vi "test Disconnect All.vi"(8 "error in (no error)":errorcluster, 11 "TestCase in":refnum<class "Switch Consumer Test Case.lvclass">) -> (0 "error out":errorcluster, 3 "TestCase out":refnum<class "Switch Consumer Test Case.lvclass">)   [LabVIEW 2017, in "Switch Consumer Test Case.lvclass"]
uses:
  Switch Consumer Test Case.lvclass
  Switch/Switch Disconnect All Message/Switch Disconnect All Message.lvclass
  C:/github/niveristand-custom-device-message-library/Source/Message/Abstract Message/Abstract Message.lvclass
  Support/Message String Action.ctl
  Switch Consumer Test Case.lvclass/Switch Consumer Test Case.ctl
  Producer/Abstract Producer/Abstract Producer.lvclass
  <vilib>/addons/_JKI Toolkits/VI Tester/TestCase.llb/TestCase.lvclass
  Consumer/Abstract Consumer/Abstract Consumer.lvclass
  C:/Program Files (x86)/National Instruments/LabVIEW 2017/vi.lib/addons/_JKI Toolkits/VI Tester/TestCase.llb/TestCase.lvclass
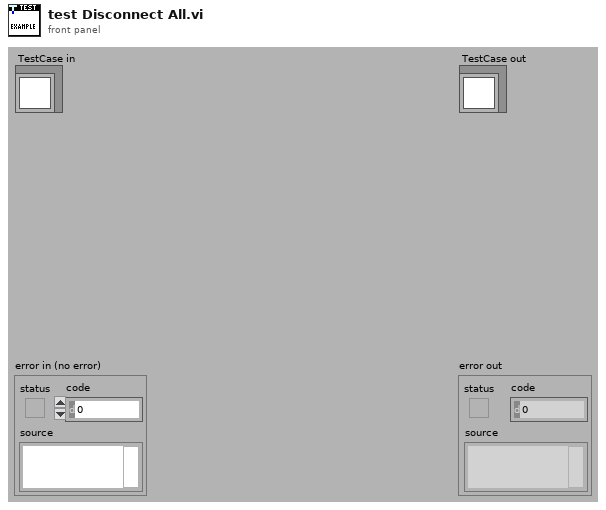
[diagram p1: front panel]
types:
  T1 = typedef "Message String Action.ctl" = enum16{"Get String", "Set String", "Reset"}
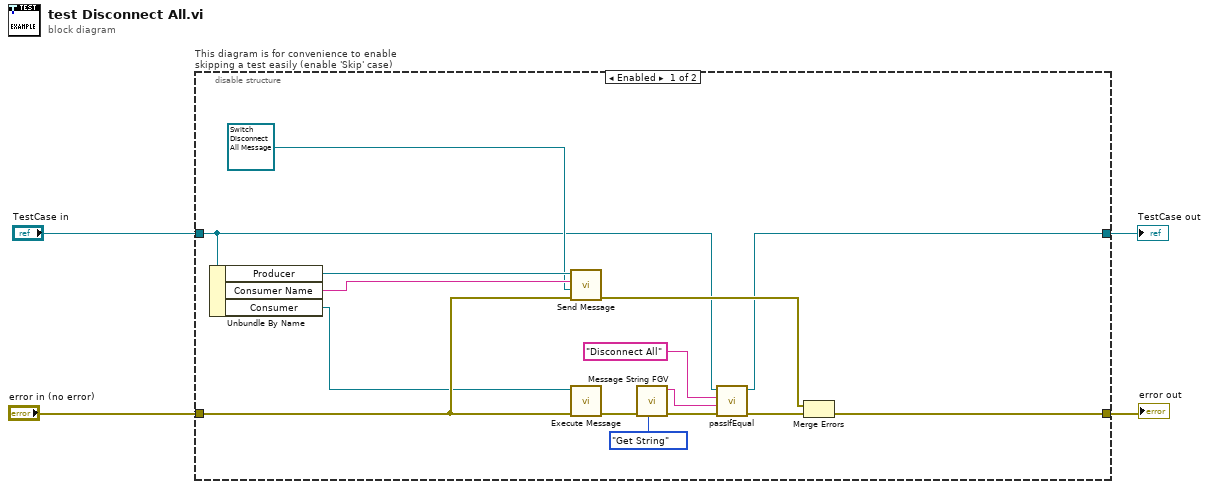
[diagram p0: block diagram]
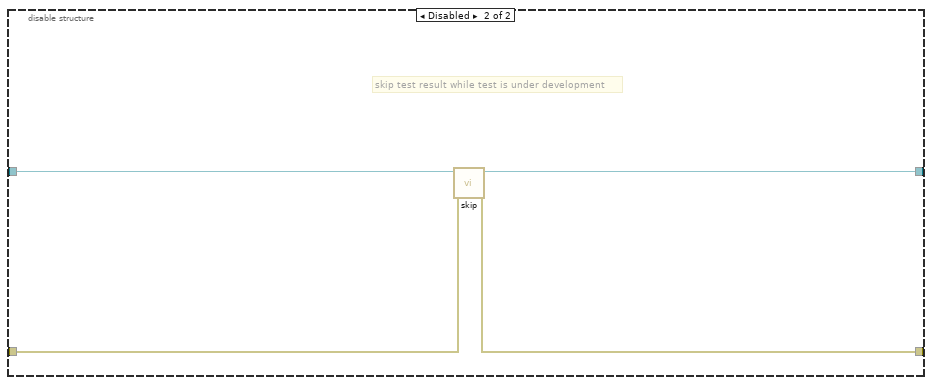
[diagram p2: hidden frame]
diagram:
  n1 = disable-structure "This diagram is for convenience to enable skipping a test easily (enable 'Skip' case)" shown="Enabled" {
    disable-tunnel: "TestCase in" -> [w7 w23]
    disable-tunnel: [w6 w21] -> w1
    disable-tunnel: [w8 w22] -> w3
    disable-tunnel: "error in (no error)" -> [w18 w20]
    frame Enabled {
      n2 = Unbundle By Name(w7) -> ("Producer"=w19:refnum<class "Abstract Producer.lvclass">, "Consumer Name"=w16:string, "Consumer"=w17:refnum<class "Abstract Consumer.lvclass">)
      n3 = call-dynamic "Send Message.vi"("error in (no error)"=w18, "Message in"=refnum<class "Switch Disconnect All Message.lvclass"> refnum ("Messaging.lvlib:Switch.lvlib:Switch Disconnect All Message.lvclass"), "Consumer in"=w16, "Abstract Producer in"=w19) -> ("error out"=w9:errorcluster)  [unwired: 5 in, 2 out]
      n4 = call "Execute Message.vi"("error in (no error)"=w18, "Abstract Consumer in"=w17) -> ("error out"=w13:errorcluster)  [unwired: 7 in, 2 out]
      n5 = call "Message String FGV.vi"("Action"=Message_String_Action."Get String", "error in (no error)"=w13) -> ("error out"=w12:errorcluster, "String out"=w11:string)  [unwired: 8 in]
      n6 = call-dynamic "passIfEqual.vi"("error in (no error)"=w12, "y"=w11, "x"="Disconnect All" ("format string"), "TestCase in"=w7) -> ("error out"=w10:errorcluster, "TestCase out"=w6:refnum<class "Switch Consumer Test Case.lvclass">)  [unwired: 6 in]
      n7 = Merge Errors(w9, w10) -> (w8:errorcluster)
    }
    frame Disabled {
      # "skip test result while test is under development"
      n8 = call <vilib>:"skip.vi"("error in (no error)"=w20, "TestCase in"=w23) -> ("error out"=w22:errorcluster, "TestCase out"=w21:refnum<class "Switch Consumer Test Case.lvclass">)  [unwired: 8 in]
    }
  }
  "error out" <- w3
  "TestCase out" <- w1
